vi "Query_SQL.vi"(4 "TypeMap":refnum<class "TypeMap.lvclass">, 5 "type":refnum<class>, 6 "commandTimeout in":i32=-1, 7 "CommandType":i32(ring)=-1 items=["Text"=1, "StoredProcedure"=4, "TableDirect"=512], 8 "error in (no error)":errorcluster, 9 "Parameters":variant, 10 "SQL Statement":string, 11 "SqlMapper in":refnum<class "SqlMapper.lvclass">) -> (0 "error out":errorcluster, 2 "Results":refnum<class>[](array[class]), 3 "SqlMapper out":refnum<class "SqlMapper.lvclass">)   [LabVIEW 2020, in "ORM_API.lvlib"]
uses:
  ORM_API.lvlib
  <vilib>/Viviota/shared/ORM.lvlibp/ORM/SqlMapper/SqlMapper.lvclass
  <vilib>/Viviota/shared/ORM.lvlibp/ORM/TypeMap/TypeMap.lvclass
  Utilities/Verify TypeMap.vi
  <vilib>/Viviota/shared/ORM.lvlibp/ORM/TypeMap/Create DynamicParameter.vi
  <userlib>/_OpenG.lib/lvdata/lvdata.llb/LVOOP Is Default Value__ogtk.vi
  <vilib>/Viviota/shared/ORM.lvlibp/ORM/TypeMap/Read TypeMap.vi
  <vilib>/Viviota/shared/ORM.lvlibp/ORM/Query Result/Next.vi
  <vilib>/Viviota/shared/ORM.lvlibp/ORM/TypeMap/ToLabVIEW_Wrap.vi
  <vilib>/Viviota/shared/ORM.lvlibp/ORM/DynamicParameters/DynamicParameters.lvclass
  <vilib>/Viviota/shared/ORM.lvlibp/ORM/Query Result/Query Result.lvclass
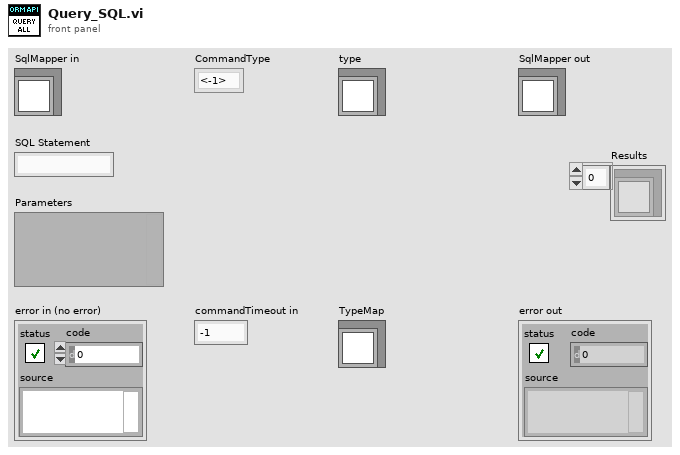
[diagram p1: front panel]
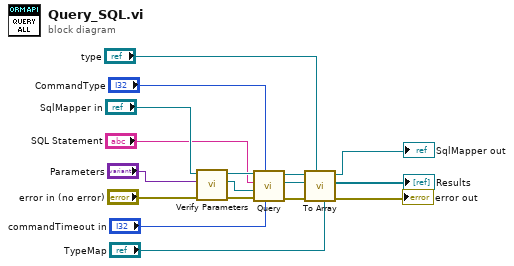
[diagram p0: block diagram]
diagram:
  n1 = call "Verify Parameters.vi"("error in (no error)"="error in (no error)", "Parameters In"="Parameters", "SqlMapper in"="SqlMapper in") -> ("error out"=w9:errorcluster, "DynamicParameters out"=w8:refnum<class "DynamicParameters.lvclass">, "SqlMapper out"=w10:refnum<class "SqlMapper.lvclass">)  [unwired: 6 in]
  n2 = call-dynamic "Query.vi"("commandTimeout"="commandTimeout in", "CommandType"="CommandType", "error in (no error)"=w9, "DynamicParameters"=w8, "sql"="SQL Statement", "SqlMapper in"=w10) -> ("error out"=w4:errorcluster, "Query Result out"=w13:refnum<class "Query Result.lvclass">, "SqlMapper out"=w12:refnum<class "SqlMapper.lvclass">)  [unwired: 3 in]
  n3 = call "To Array.vi"("TypeMap"="TypeMap", "Type"="type", "error in (no error)"=w4, "Query Result in"=w13, "SqlMapper in"=w12) -> ("error out"=→"error out":errorcluster, "Array"=→"Results":refnum<class>[], "SqlMapper out"=→"SqlMapper out":refnum<class "SqlMapper.lvclass">)  [unwired: 4 in]
